vi "LEP_RV_TargetTemplateVersion.vi"(8 "error in (no error)":errorcluster, 11 "Path":path) -> (0 "error out":errorcluster, 2 "Version":string, 3 "Path plus Version":path)   [LabVIEW 2011]
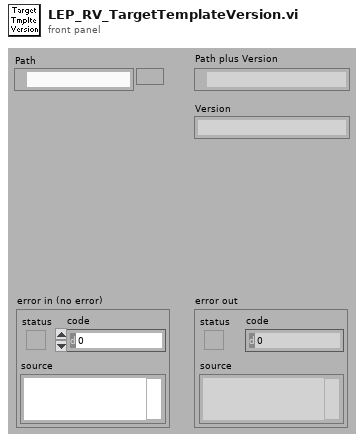
[diagram p1: front panel]
types:
  T1 = cluster{"KEIL Path":path, "Port Range Start":u16, "Port Range End":u16, "UV IP Address":string}
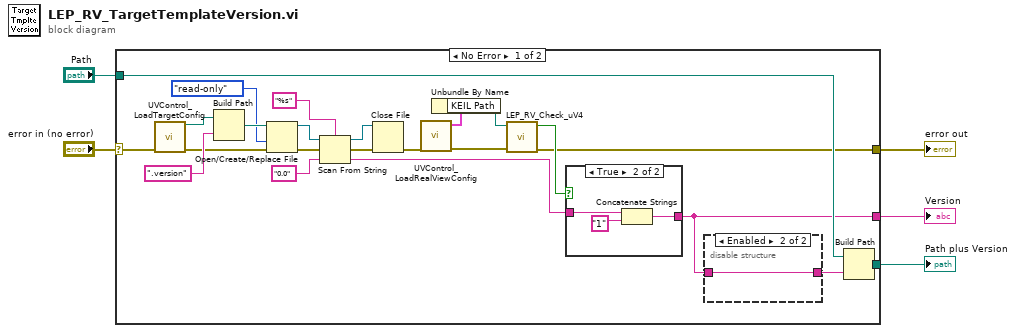
[diagram p0: block diagram]
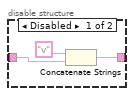
[diagram p3: hidden frame]
diagram:
  n1 = case shown="No Error" "error in (no error)" {
    selector: "error in (no error)" -> [w14 w37]
    tunnel: [w12 w37] -> w4
    tunnel: [w15 _] -> w3
    tunnel: [w10 _] -> w2
    tunnel: "Path" -> [w16 _]
    frame No Error {
      n2 = call "UVControl_LoadTargetConfig.vi"("error in (no error)"=w14) -> ("Target Template Path"=w28:path, "error out"=w26:errorcluster)  [unwired: 9 in, 4 out]
      n3 = Build Path(base path=w28, name or relative path=".version") -> (appended path=w25:path)
      n4 = Open/Create/Replace File(file path (use dialog)=w25, error in=w26, access (0:read/write)=enum16{"read/write", "read-only", "write-only"}."read-only") -> (refnum out=w23:refnum<file>, error out=w22:errorcluster)  [unwired: 3 in, 1 out]
      n5 = Scan From String("%s" ("format string"), w23, w22, default 1="0.0" ("default value 1")) -> (w19:refnum<file>, w18:errorcluster, output 1=w11:string)
      n6 = Close File(refnum=w19, error in=w18) -> (error out=w8:errorcluster)  [unwired: 1 out]
      n7 = call "UVControl_LoadRealViewConfig.vi"("error in (no error)"=w8) -> ("uVisionConfig"=w9:T1, "error out"=w7:errorcluster)  [unwired: 11 in, 2 out]
      n8 = Unbundle By Name(w9) -> ("KEIL Path"=w6:path)
      n9 = call "LEP_RV_Check_uV4.vi"("error in (no error)"=w7, "KEIL Path"=w6) -> ("error out"=w12:errorcluster, "uv4 installed"=w13:bool)  [unwired: 8 in]
      n10 = case shown="True" w13 {
        tunnel: w11 -> [w29 w32]
        tunnel: [w29 w30] -> w10
        frame False {
        }
        frame True {
          n11 = Concatenate Strings(w32, "1" ("string")) -> (w30:string)
        }
      }
      n12 = disable-structure shown="Enabled" {
        disable-tunnel: w10 -> [w35 w36]
        disable-tunnel: [w33 w36] -> w17
        frame Disabled {
          n13 = Concatenate Strings("v" ("string"), w35) -> (w33:string)
        }
        frame Enabled {
        }
      }
      n14 = Build Path(base path=w16, name or relative path=w17) -> (appended path=w15:path)
    }
    frame Error {
    }
  }
  "error out" <- w4
  "Path plus Version" <- w3
  "Version" <- w2
